vi "Reset Buffer.vi"(8 "error in (no error)":errorcluster, 11 "RTL-SDR in":refnum<class "RTL-SDR.lvclass">) -> (0 "error out":errorcluster, 1 "function return":i32, 3 "RTL-SDR out":refnum<class "RTL-SDR.lvclass">)   [LabVIEW 2015, in "RTL-SDR.lvclass"]
doc: "Created IvanLis by LabVIEW Portal\nProfile: http://labviewportal.org/memberlist.php?mode=viewprofile&u=987\neMail: IvanLisanov@gMail.com\nTelegram: https://t.me/IvanLis"
uses:
  RTL-SDR.lvclass
  RTL-SDR.lvclass/RTL-SDR.ctl
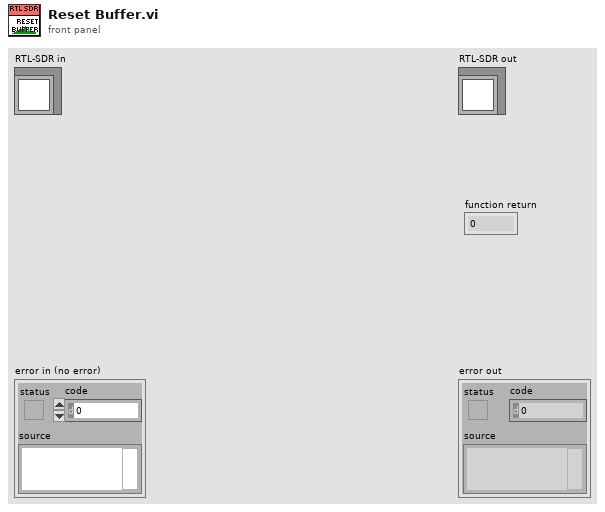
[diagram p1: front panel]
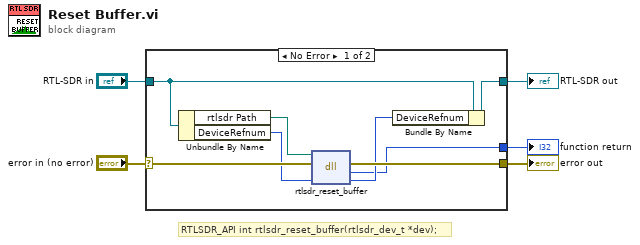
[diagram p0: block diagram]
diagram:
  # "RTLSDR_API int rtlsdr_reset_buffer(rtlsdr_dev_t *dev);"
  n1 = case shown="No Error" "error in (no error)" {
    selector: "error in (no error)" -> [w13 w15]
    tunnel: [w12 w15] -> w4
    tunnel: [w11 w14] -> w2
    tunnel: "RTL-SDR in" -> [w9 w14]
    tunnel: [w6 _] -> w1
    frame No Error {
      n2 = Unbundle By Name(w9) -> ("rtlsdr Path"=w7:path, "DeviceRefnum"=w8:u64)
      n3 = dll-call lib="C:/Users/Ivan/Desktop/D-23-09-24 (RTL-SDR)/Project (Pelleng-SDR)/rtlsdr/dll/rtlsdr.*" fn="rtlsdr_reset_buffer"(path in=w7, error in=w13, "DeviceRefnum"=w8) -> (error out=w12:errorcluster, "return type"=w6:i32, "DeviceRefnum"=w10:u64)  [unwired: 1 in, 1 out]
      n4 = Bundle By Name(cluster=w9, "DeviceRefnum"=w10) -> (w11:refnum<class "RTL-SDR.lvclass">)
    }
    frame Error {
    }
  }
  "error out" <- w4
  "RTL-SDR out" <- w2
  "function return" <- w1
